vi "Test Pick and Replace.vi"() -> ()   [LabVIEW 2011]
uses:
  WorkTable Class/Type Definitions/Worktable_Mode.ctl
  Config Manager Class/Type Definitions/Fiducial Type.ctl
  Config Manager Class/Type Definitions/Part Type.ctl
  Gantry Class/Gantry Class.lvclass
  WorkTable Class/WorkTable Class.lvclass
  Vec3d Class/Vec3d Class.lvclass
  CameraTool Class/CameraTool Class.lvclass
  PickerTool Class.lvclass
  Gantry Application/Procedure Classes/Potting Procedure/Potting Procedure.lvclass
  Config Manager Class/Config Manager Class.lvclass
panel:
  in  "stop":bool
  out "results":string
  in  "Slot":i32
  in  "Chuck":i32=4
  in  "Config Folder":path=path "C:/Users/husker/Desktop/gantry/Config"
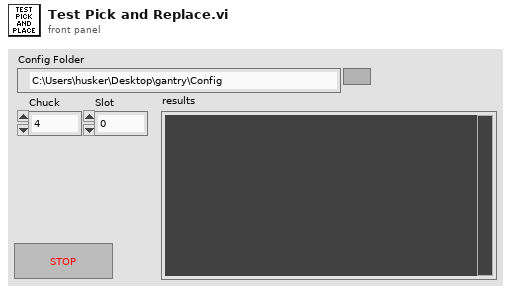
[diagram p1: front panel]
types:
  T1 = typedef "Fiducial Type.ctl" = enum16{"HDI", "BBM"}
  T2 = typedef "Worktable_Mode.ctl" = enum16{"Encapsulation", "Gluing"}
  T3 = cluster{"Feature Coordinates":refnum<class "Vec3d Class.lvclass">, "Feature Name":string}[]
  T4 = typedef "Worktable_Module Slot.ctl" = cluster{"Slot State":enum16{"Empty", "Unglued", "Stamped", "PartOnTop", "Weighted", "Unpotted", "Potted"}, "BBM Type":enum16{"None", "BBM", "GlassSlide"}, "HDI Type":enum16{"None", "HDI", "Polyimide"}, "Vacuum Channel":u8, "Location/Orientation BBM":T5, "Location/Orientation HDI":T5, "S/N":string}
  T5 = typedef "Position_Orientation.ctl" = cluster{"Center":refnum<class "Vec3d Class.lvclass">, "Orientation":refnum<class "Orient3d Class.lvclass">}
  T6 = typedef "Part Type.ctl" = enum16{"BBM", "HDI", "BARE HDI", "GLUERESERVOIR", "STAMP_1", "STAMP_2", "STAMP_3", "STAMP_4", "STAMP_5", "WEIGHT_1", "WEIGHT_2", "WEIGHT_3", "WEIGHT_4", "WEIGHT_5", "WEIGHT_6", "WEIGHT_7", "WEIGHT_8", "PICKER_TOOL", "GRABER_TOOL"}
  T7 = typedef "Fiducial Image.ctl" = cluster{"Fiducial Image":T8, "Selected Fiducial":T10, "fiducial name":string}
  T8 = typedef "Physical Image.ctl" = cluster{"Image Position":refnum<class "Vec3d Class.lvclass">, "Image Reference":T9, "Field of View":cluster{"x(mm)":dbl, "y(mm)":dbl}}
  T9 = typedef "IMAQ Image.ctl" = refnum<image>
  T10 = typedef "Fiducial with Source.ctl" = cluster{"Fiducial Image Coordinate":refnum<class "Vec3d Class.lvclass">, "Fiducial Source":enum16{"Pattern Recognition", "User", "Error", "Default"}}
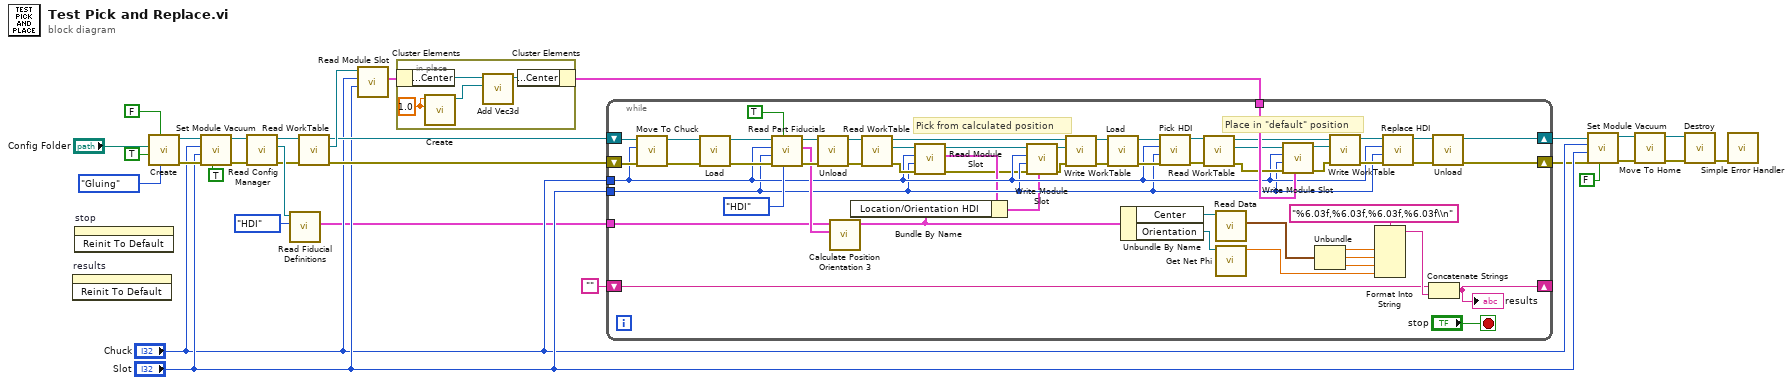
[diagram p0: block diagram]
diagram:
  n1 = invoke on="results" class="Str" method="Reinit To Default"() -> ()  [unwired: 3 in, 3 out]
  n2 = invoke on="stop" class="Bool" method="Reinit To Default"() -> ()  [unwired: 3 in, 3 out]
  n3 = call "Create.vi"("Worktable Mode"=Worktable_Mode."Gluing", "Virtual Mode"=FALSE, "HOME?"=TRUE, "Config Folder"="Config Folder") -> ("error out"=w23:errorcluster, "Gantry out"=w24:refnum<class "Gantry Class.lvclass">)  [unwired: 6 in]
  n4 = call-dynamic "Set Module Vacuum.vi"("On/Off"=TRUE, "error in"=w23, "Slot Number"="Slot", "Chuck Number"="Chuck", "Gantry in"=w24) -> ("error out"=w18:errorcluster, "Gantry out"=w19:refnum<class "Gantry Class.lvclass">)  [unwired: 5 in]
  n5 = call-dynamic "Read Config Manager.vi"("error in"=w18, "Gantry in"=w19) -> ("error out"=w9:errorcluster, "Config Manager"=w27:refnum<class "Config Manager Class.lvclass">, "Gantry out"=w12:refnum<class "Gantry Class.lvclass">)  [unwired: 7 in]
  n6 = call "Read Fiducial Definitions.vi"("Fiducial Type"=Fiducial_Type."HDI", "Config Manager in"=w27) -> ("Feature Definitions"=w2:T3)  [unwired: 7 in, 2 out]
  n7 = call-dynamic "Read WorkTable.vi"("error in"=w9, "Gantry Class in"=w12) -> ("error out"=w8:errorcluster, "WorkTable Class.lvclass"=w11:refnum<class "WorkTable Class.lvclass">, "Gantry Class out"=w10:refnum<class "Gantry Class.lvclass">)  [unwired: 7 in]
  n8 = call-dynamic "Read Module Slot.vi"("slot"="Slot", "chuck"="Chuck", "WorkTable in"=w11) -> ("Module Slot"=w13:T4)  [unwired: 6 in, 2 out]
  n9 = in-place {
    w34 = 1.0 ("Y")
    n10 = in-place-cluster #1(w13) -> ("Location/Orientation HDI.Center"=w33:refnum<class "Vec3d Class.lvclass">)
    n11 = call "Create.vi"("Y"=w34, "X"=w34) -> ("Vec3d Class out"=w32:refnum<class "Vec3d Class.lvclass">)  [unwired: 8 in, 1 out]
    n12 = call-dynamic "Add Vec3d.vi"(10:"Vec3d Class in"=w32, 11:"Vec3d Class in"=w33) -> ("Vec3d Class out"=w31:refnum<class "Vec3d Class.lvclass">)  [unwired: 8 in, 1 out]
    n13 = in-place-cluster #1("Location/Orientation HDI.Center"=w31) -> (w6:T4)
  }
  n14 = while {
    tunnel: "Chuck" -> [w41]
    tunnel: "Slot" -> [w40]
    tunnel: w6 -> [w72]
    shift-right: [w66] -> w4
    shift-left: w10 -> [w74]
    shift-right: [w65] -> w3
    shift-left: w8 -> [w73]
    tunnel: w2 -> [w61]
    shift-right: [w52] -> _
    shift-left: "" -> [w53]
    stop <- "stop" stop-if-true
    # "Place in \"default\" position"
    # "Pick from calculated position"
    n15 = call-dynamic "Move To Chuck.vi"("error in"=w73, "Chuck"=w41, "Gantry in"=w74) -> ("error out"=w79:errorcluster, "Gantry out"=w80:refnum<class "Gantry Class.lvclass">)  [unwired: 7 in]
    n16 = call "Load.vi"("error in"=w79, "Gantry In"=w80) -> ("error out"=w89:errorcluster, "CameraTool out"=w90:refnum<class "CameraTool Class.lvclass">)  [unwired: 8 in]
    n17 = call-dynamic "Read Part Fiducials.vi"("Part Type"=Part_Type."HDI", "Dispose Images?"=TRUE, "error in"=w89, "Slot"=w40, "Chuck"=w41, "CameraTool in"=w90) -> ("error out"=w81:errorcluster, "Fiducials"=w62:T7[], "CameraTool out"=w82:refnum<class "CameraTool Class.lvclass">)  [unwired: 3 in]
    n18 = call "Unload.vi"("error in"=w81, "CameraTool in"=w82) -> ("error out"=w46:errorcluster, "Gantry out"=w48:refnum<class "Gantry Class.lvclass">)  [unwired: 8 in]
    n19 = call "Calculate Position Orientation 3.vi"("Fiducials"=w62, "Feature Definitions"=w61) -> ("PositionOrientation"=w38:T5)  [unwired: 8 in, 1 out]
    n20 = call-dynamic "Read WorkTable.vi"("error in"=w46, "Gantry Class in"=w48) -> ("error out"=w42:errorcluster, "WorkTable Class.lvclass"=w45:refnum<class "WorkTable Class.lvclass">, "Gantry Class out"=w49:refnum<class "Gantry Class.lvclass">)  [unwired: 7 in]
    n21 = call-dynamic "Read Module Slot.vi"("error in"=w42, "slot"=w40, "chuck"=w41, "WorkTable in"=w45) -> ("error out"=w35:errorcluster, "Module Slot"=w39:T4, "WorkTable out"=w36:refnum<class "WorkTable Class.lvclass">)  [unwired: 5 in]
    n22 = Bundle By Name(cluster=w39, "Location/Orientation HDI"=w38) -> (w37:T4)
    n23 = call-dynamic "Write Module Slot.vi"("Module Slot"=w37, "error in"=w35, "slot"=w40, "chuck"=w41, "WorkTable in"=w36) -> ("error out"=w44:errorcluster, "WorkTable out"=w50:refnum<class "WorkTable Class.lvclass">)  [unwired: 5 in]
    n24 = call-dynamic "Write WorkTable.vi"("error in (no error)"=w44, "WorkTable Class.lvclass"=w50, "Gantry Class in"=w49) -> ("error out"=w43:errorcluster, "Gantry Class out"=w47:refnum<class "Gantry Class.lvclass">)  [unwired: 7 in]
    n25 = call "Load.vi"("error in"=w43, "Gantry in"=w47) -> ("error out"=w86:errorcluster, "PickerTool out"=w85:refnum<class "PickerTool Class.lvclass">)  [unwired: 8 in]
    n26 = Unbundle By Name(w38) -> ("Center"=w63:refnum<class "Vec3d Class.lvclass">, "Orientation"=w64:refnum<class "Orient3d Class.lvclass">)
    n27 = call-dynamic "Pick HDI.vi"("error in"=w86, "Slot"=w40, "Chuck"=w41, "PickerTool in"=w85) -> ("error out"=w70:errorcluster, "PickerTool out"=w71:refnum<class "PickerTool Class.lvclass">)  [unwired: 6 in]
    n28 = call-dynamic "Read WorkTable.vi"("error in"=w70, "Gantry Class in"=w71) -> ("error out"=w67:errorcluster, "WorkTable Class.lvclass"=w68:refnum<class "WorkTable Class.lvclass">, "Gantry Class out"=w69:refnum<class "PickerTool Class.lvclass">)  [unwired: 7 in]
    n29 = call-dynamic "Read Data.vi"("Vec3d Class in"=w63) -> ("Data"=w59:cluster{"X":dbl, "Y":dbl, "Z":dbl})  [unwired: 8 in, 2 out]
    n30 = call "Get Net Phi.vi"("Orient3d"=w64) -> ("phi(deg)"=w55:dbl)  [unwired: 8 in, 2 out]
    n31 = call-dynamic "Write Module Slot.vi"("Module Slot"=w72, "error in"=w67, "slot"=w40, "chuck"=w41, "WorkTable in"=w68) -> ("error out"=w77:errorcluster, "WorkTable out"=w78:refnum<class "WorkTable Class.lvclass">)  [unwired: 5 in]
    n32 = Unbundle(w59) -> ("X"=w58:dbl, "Y"=w57:dbl, "Z"=w56:dbl)
    n33 = call-dynamic "Write WorkTable.vi"("error in (no error)"=w77, "WorkTable Class.lvclass"=w78, "Gantry Class in"=w69) -> ("error out"=w75:errorcluster, "Gantry Class out"=w76:refnum<class "PickerTool Class.lvclass">)  [unwired: 7 in]
    n34 = Format Into String(format string="%6.03f,%6.03f,%6.03f,%6.03f\\n", w58, w57, w56, w55) -> (resulting string=w54:string)  [unwired: 2 in, 1 out]
    n35 = call-dynamic "Replace HDI.vi"("error in"=w75, "Slot"=w40, "Chuck"=w41, "PickerTool in"=w76) -> ("error out"=w84:errorcluster, "PickerTool out"=w83:refnum<class "PickerTool Class.lvclass">)  [unwired: 6 in]
    n36 = Concatenate Strings(w53, w54) -> (w52:string)
    "results" <- w52
    n37 = call "Unload.vi"("error in"=w84, "PickupTool in"=w83) -> ("error out"=w65:errorcluster, "Gantry out"=w66:refnum<class "Gantry Class.lvclass">)  [unwired: 8 in]
  }
  n38 = call-dynamic "Set Module Vacuum.vi"("On/Off"=FALSE, "error in"=w3, "Slot Number"="Slot", "Chuck Number"="Chuck", "Gantry in"=w4) -> ("error out"=w16:errorcluster, "Gantry out"=w17:refnum<class "Gantry Class.lvclass">)  [unwired: 5 in]
  n39 = call-dynamic "Move To Home.vi"("error in"=w16, "Gantry in"=w17) -> ("error out"=w15:errorcluster, "Gantry out"=w14:refnum<class "Gantry Class.lvclass">)  [unwired: 8 in]
  n40 = call "Destroy.vi"("error in"=w15, "Gantry Class in"=w14) -> ("error out"=w20:errorcluster)  [unwired: 9 in]
  n41 = call <vilib>:"Simple Error Handler.vi"("error in (no error)"=w20) -> ()  [unwired: 4 in, 5 out]
